vi "counter.vi"() -> ()   [LabVIEW 2012]
uses:
  <vilib>/addons/internet/NI_InternetTK_Core_VIs.lvlib
panel:
  in  "Relative Counter Path":path=path "../counter.txt"
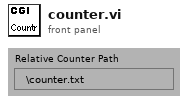
[diagram p1: front panel]
types:
  T1 = typedef "CGI Connection Info.ctl" = cluster{"name":string, "type":T2, "session":T3}
  T2 = typedef "CGI Request Type.ctl" = enum16{"cgi", ".spool first", ".spool", ".spool last"}
  T3 = typedef "HTTP Session.ctl" = refnum<k1>
  T4 = typedef "NI_FTP.lvlib/Keyed Array.ctl" = cluster{"keys":string[], "values":string[]}
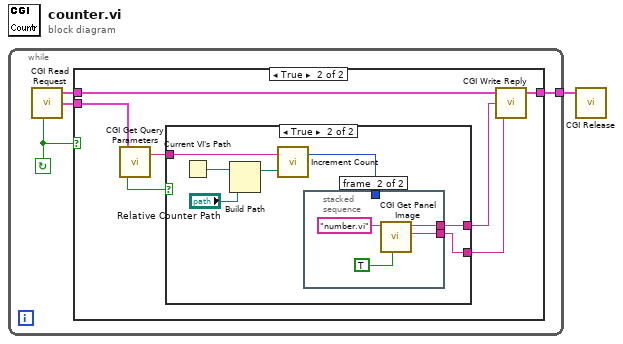
[diagram p0: block diagram]
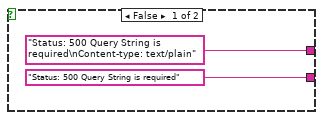
[diagram p3: hidden frame]
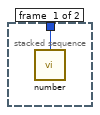
[diagram p4: hidden frame]
diagram:
  n1 = while {
    tunnel: [w5] -> w1
    stop <- w2 continue-if-true
    n2 = call <vilib>:"CGI Read Request.vi"() -> ("valid request?"=w2:bool, "cgi connection info"=w4:T1, "env"=w3:T4)  [unwired: 4 in, 1 out]
    n3 = case shown="True" w2 {
      tunnel: [w6 w11] -> w5
      tunnel: w4 -> [w6 w10]
      tunnel: w3 -> [_ w9]
      frame False {
      }
      frame True {
        n4 = call <vilib>:"CGI Get Query Parameters.vi"("env"=w9) -> ("query string"=w8:string, "has query string"=w7:bool)  [unwired: 1 out]
        n5 = case shown="True" w7 {
          tunnel: w8 -> [_ w20]
          tunnel: ["Status: 500 Query String is required" ("content") w17] -> w12
          tunnel: ["Status: 500 Query String is required\nContent-type: text/plain" w16] -> w13
          frame False {
          }
          frame True {
            n6 = Current VI's Path() -> (path=w21:path)
            n7 = Build Path(base path=w21, name or relative path="Relative Counter Path") -> (appended path=w18:path)
            n8 = call "Increment Count.vi"("file path"=w18, "token"=w20) -> ("count"=w19:i32)  [unwired: 1 in]
            n9 = stacked-sequence {
              tunnel: w19 -> [w23 _]
              tunnel: [_ w25] -> w17
              tunnel: [_ w24] -> w16
              frame #0 {
                n10 = call "number.vi"(w23) -> ()
              }
              frame #1 {
                n11 = call <vilib>:"CGI Get Panel Image.vi"("entire panel (F)"=TRUE ("Entire Panel (F)"), "vi name"="number.vi" ("VI name")) -> ("content"=w25:string, "content header"=w24:string)  [unwired: 7 in, 1 out]
              }
            }
          }
        }
        n12 = call <vilib>:"CGI Write Reply.vi"("content"=w12, "header"=w13, "cgi connection info"=w10) -> ("cgi connection info out"=w11:T1)  [unwired: 2 in]
      }
    }
  }
  n13 = call <vilib>:"CGI Release.vi"("cgi connection info"=w1) -> ()  [unwired: 5 in]
